vi "Read Frequency (Hz).vi"(8 "error in (no error)":errorcluster, 11 "SAM in":refnum<class "SAM.lvclass">) -> (0 "error out":errorcluster, 2 "Frequency (Hz)":dbl, 3 "SAM out":refnum<class "SAM.lvclass">)   [LabVIEW 2020, in "SAM.lvclass"]
uses:
  SAM.lvclass
  SAM.lvclass/SAM.ctl
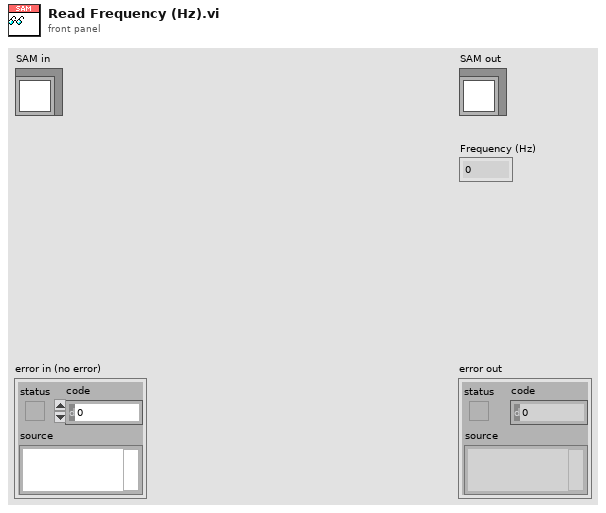
[diagram p1: front panel]
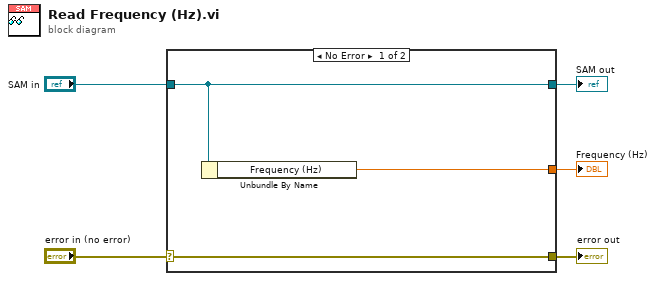
[diagram p0: block diagram]
diagram:
  n1 = case shown="No Error" "error in (no error)" {
    selector: "error in (no error)" -> [w8 w9]
    tunnel: [w8 w9] -> w4
    tunnel: [w7 w10] -> w2
    tunnel: "SAM in" -> [w7 w10]
    tunnel: [w6 _] -> w1
    frame No Error {
      n2 = Unbundle By Name(w7) -> ("Frequency (Hz)"=w6:dbl)
    }
    frame Error {
    }
  }
  "error out" <- w4
  "SAM out" <- w2
  "Frequency (Hz)" <- w1
